vi "Event Log.Debug Util, Print to File.vi"(5 "Close":bool, 7 "Enable":bool=TRUE, 10 "Messages":string[](array[string]), 11 "Message":string) -> ()   [LabVIEW 2024, in "EQMF.lvlib" / "Event Log.lvlib"]
uses:
  Event Log.lvlib
  <vilib>/Utility/sysdir.llb/System Directory Type.ctl
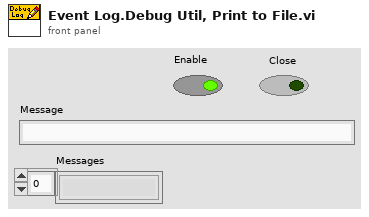
[diagram p1: front panel]
types:
  T1 = enum16{"open", "replace", "create", "open or create", "replace or create", "replace or create with confirmation"}
  T2 = typedef "System Directory Type.ctl" = i32
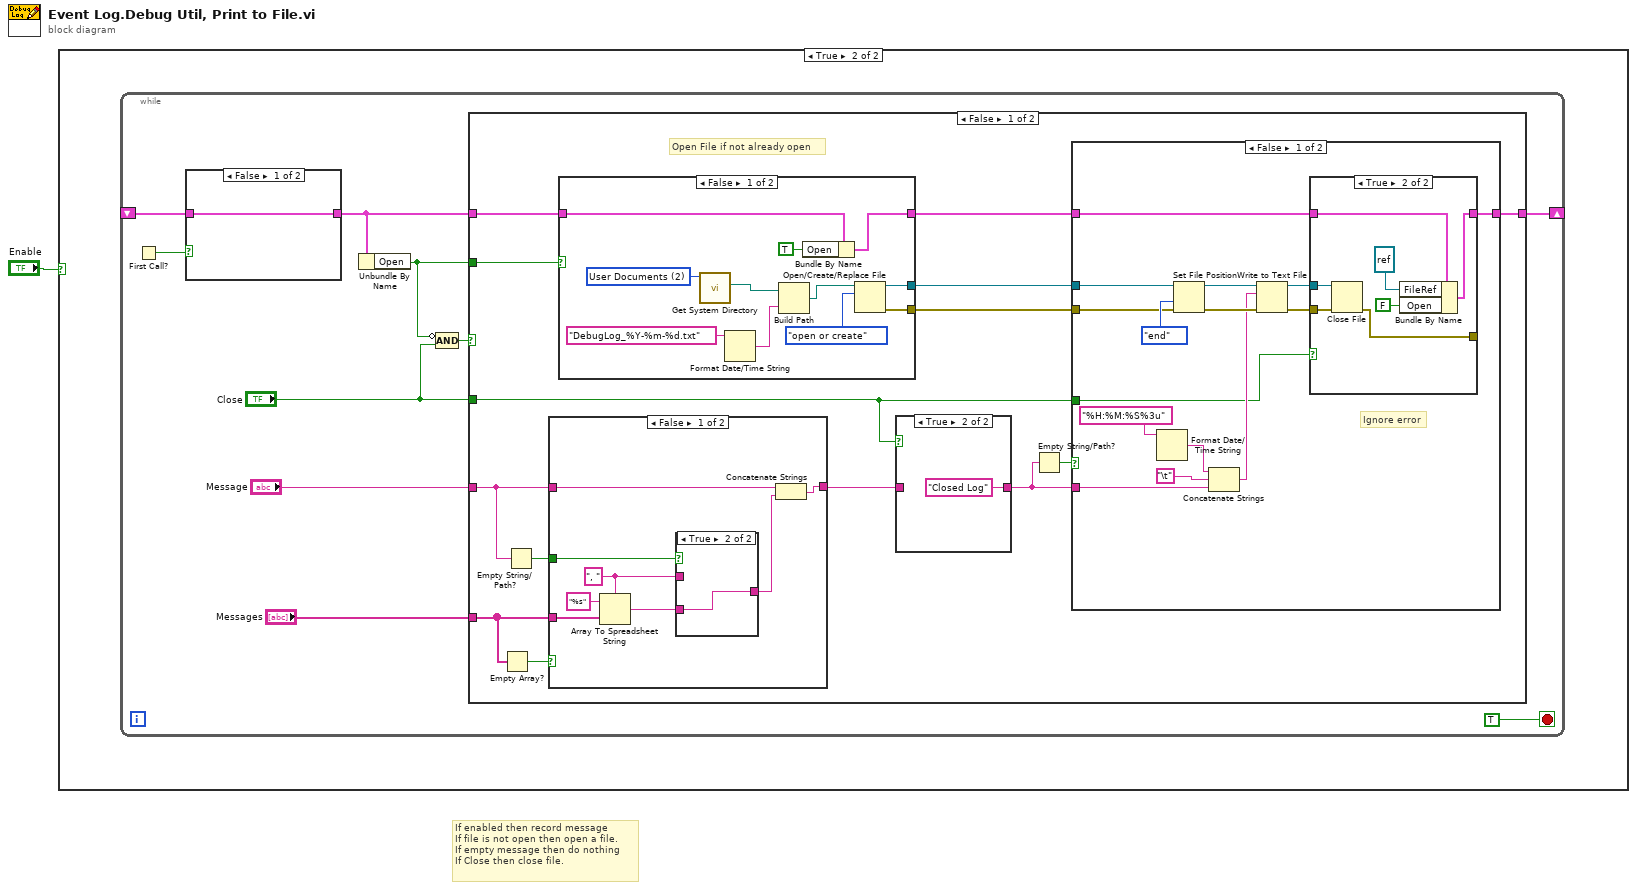
[diagram p0: block diagram]
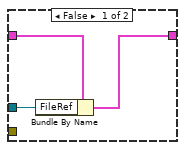
[diagram p4: hidden frame]
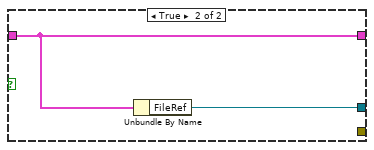
[diagram p6: hidden frame]
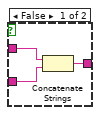
[diagram p7: hidden frame]
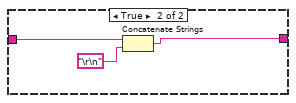
[diagram p8: hidden frame]
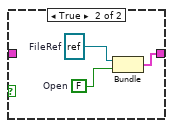
[diagram p10: hidden frame]
diagram:
  # "If enabled then record message\nIf file is not open then open a file.\nIf empty message then do nothing\nIf Close then close file."
  n1 = case shown="True" "Enable" {
    frame False {
    }
    frame True {
      n2 = while {
        shift-right: [w6] -> _
        shift-left: _ -> [w10]
        stop <- TRUE stop-if-true
        n3 = First Call?() -> (First Call?: T/F=w11:bool)
        n4 = case shown="False" w11 {
          tunnel: w10 -> [w83 _]
          tunnel: [w83 w84] -> w8
          frame False {
          }
          frame True {
            w86 = FALSE  # Open
            w85 = refnum<file> refnum  # FileRef
            n5 = Bundle("FileRef"=w85, "Open"=w86) -> (w84:cluster{"FileRef":refnum<file>, "Open":bool})  [unwired: 1 in]
          }
        }
        n6 = Unbundle By Name(w8) -> ("Open"=w4:bool)
        n7 = Compound Arithmetic op=AND(invert w4, "Close") -> (w2:bool)
        n8 = case shown="False" w2 {
          tunnel: "Messages" -> [w25 _]
          tunnel: w4 -> [w22 _]
          tunnel: w8 -> [w21 w82]
          tunnel: [w17 w82] -> w6
          tunnel: "Message" -> [w13 _]
          tunnel: "Close" -> [w16 _]
          frame False {
            # "Open File if not already open"
            n9 = Empty Array?(array=w25) -> (empty?=w24:bool)
            n10 = Empty String/Path?(string/path=w13) -> (empty?=w23:bool)
            n11 = case shown="False" w24 {
              tunnel: w25 -> [w73 _]
              tunnel: w23 -> [w71 _]
              tunnel: w13 -> [w68 w81]
              tunnel: [w69 w79] -> w12
              frame False {
                w72 = ", " ("format string")
                n12 = Array To Spreadsheet String(delimiter (Tab)=w72, array=w73, 3:"%s" ("format string")) -> (spreadsheet string=w70:string)
                n13 = case shown="True" w71 {
                  tunnel: w72 -> [w77 _]
                  tunnel: w70 -> [w76 w78]
                  tunnel: [w75 w78] -> w67
                  frame False {
                    n14 = Concatenate Strings(w77, w76) -> (w75:string)
                  }
                  frame True {
                  }
                }
                n15 = Concatenate Strings(w68, w67) -> (w69:string)
              }
              frame True {
                n16 = Concatenate Strings(w81, "\r\n") -> (w79:string)
              }
            }
            n17 = case shown="False" w22 {
              tunnel: w21 -> [w56 w65]
              tunnel: [w57 w65] -> w18
              tunnel: [w59 w66] -> w20
              tunnel: [w58 _] -> w19
              frame False {
                w64 = T2 2 items=["User Home"=0, "User Desktop"=1, "User Documents"=2, "User Application Data"=3, "User Preferences"=4, "User Temporary"=5, "Public Documents"=6, "Public Application Data"=7, "Public Preferences"=8, "Public Cache"=13, "System Core Libraries"=9, "System Installed Libraries"=10, "Application Files"=11, "Boot Volume Root"=12] ("system directory type")
                n18 = call <vilib>:"Get System Directory.vi"("system directory type"=w64) -> ("system directory"=w54:path)  [unwired: 10 in]
                n19 = Format Date/Time String(time format string (%c)="DebugLog_%Y-%m-%d.txt") -> (date/time string=w60:string)  [unwired: 2 in]
                n20 = Build Path(base path=w54, name or relative path=w60) -> (appended path=w62:path)
                n21 = Bundle By Name(cluster=w56, "Open"=TRUE) -> (w57:cluster{"FileRef":refnum<file>, "Open":bool})
                n22 = Open/Create/Replace File(file path (use dialog)=w62, operation (0:open)=T1."open or create") -> (refnum out=w59:refnum<file>, error out=w58:errorcluster)  [unwired: 4 in, 1 out]
              }
              frame True {
                n23 = Unbundle By Name(w65) -> ("FileRef"=w66:refnum<file>)
              }
            }
            n24 = case shown="True" w16 {
              tunnel: w12 -> [w26 _]
              tunnel: [w26 "Closed Log"] -> w15
              frame False {
              }
              frame True {
              }
            }
            n25 = Empty String/Path?(string/path=w15) -> (empty?=w14:bool)
            n26 = case shown="False" w14 {
              tunnel: w20 -> [w39 _]
              tunnel: w19 -> [w38 _]
              tunnel: w18 -> [w35 w53]
              tunnel: [w32 w53] -> w17
              tunnel: w15 -> [w31 _]
              tunnel: w16 -> [w29 _]
              frame False {
                # "Ignore error"
                n27 = Format Date/Time String(time format string (%c)="%H:%M:%S%3u") -> (date/time string=w41:string)  [unwired: 2 in]
                n28 = Set File Position(refnum=w39, from (0:start)=enum16{"start", "end", "current"}."end", error in=w38) -> (refnum out=w37:refnum<file>, error out=w36:errorcluster)  [unwired: 1 in]
                n29 = Concatenate Strings(w41, "\t", w31) -> (w33:string)
                n30 = Write to Text File(file (use dialog)=w37, text=w33, error in=w36) -> (refnum out=w34:refnum<file>, error out=w30:errorcluster)  [unwired: 1 in, 1 out]
                n31 = case shown="True" w29 {
                  tunnel: w35 -> [w45 w52]
                  tunnel: w34 -> [w44 w50]
                  tunnel: [w43 w47] -> w32
                  tunnel: w30 -> [_ w51]
                  tunnel: [_ w46] -> _
                  frame False {
                    n32 = Bundle By Name(cluster=w45, "FileRef"=w44) -> (w43:cluster{"FileRef":refnum<file>, "Open":bool})
                  }
                  frame True {
                    n33 = Close File(refnum=w50, error in=w51) -> (error out=w46:errorcluster)  [unwired: 1 out]
                    n34 = Bundle By Name(cluster=w52, "FileRef"=refnum<file> refnum, "Open"=FALSE) -> (w47:cluster{"FileRef":refnum<file>, "Open":bool})
                  }
                }
              }
              frame True {
              }
            }
          }
          frame True {
            # "Do nothing\nClosed before was opened."
          }
        }
      }
    }
  }
